vi "Window1.vi"() -> ()   [LabVIEW 8.6]
uses:
  user32.dll
  EventHandlerEnum.ctl
  Engines/SettingsEngine/SettingsEngineEnum.ctl
  <vilib>/Instr/_visa.llb/VISA Set IO Buffer Mask.ctl
  <vilib>/Instr/_visa.llb/VISA Configure Serial Port (Instr).vi
panel:
  in  "Tab Control":enum32{"Main", "Setup", "Debug Data"}(tab)
  in  "FPV View":bool
  out "Climb Rate":sgl(knob) scale=-5.0..5.0 scale format="%#.2g"
  out "Course/Bearing":cluster{i16, i16}(knob) scale=0.0..360.0 scale format="%.0f°"
  out "Altitude":cluster{i32, i32}(knob) scale=0.0..200.0
  out "Air Speed":cluster{i16, i16}(knob)={0, 31} scale=0.0..40.0
  out "UAV Longitude 2":dbl format="%.6g°"
  out "Est Time Left":i32
  out "Current WP":i32
  out "Amps":i32
  out "Watts":i32
  out "Throttle":dbl(slide) scale=0.0..100.0
  out "Battery":dbl(slide) scale=0.0..10.0
  out "Pitch":i32
  out "Roll":i32
  out "Nav Display":picture
  out "Distance to WP":i32 format="%.0f m"
  out "Ground Speed":i32 format="%.0f m/s"
  out "Air Speed":i32 format="%.0f m/s"
  out "UAV Longitude":dbl format="%.6g°"
  out "UAV Latitude":dbl format="%.6g°"
  in  "Stop":bool
  in  "WebBrowser":refnum<k7>(container)
  out "StreamingProgressPercentage":i32(slide) scale=0.0..100.0
  out "Baud Rate":string(combo)="9600"
  out "COM Port":refnum<visa-resource-name>
  out "Camera Position 2":T1
  out "Version":string
  out "VersionAppType":i32(ring) items=["EnterpriseClientGE", "ProGE", "PlusGE", "FreeGE", "UnknownGE"]
  out "ElevationExaggeration":dbl
  in  "Set":bool
  in  "AutoPilotSpeed":dbl=0.5
  in  "Camera Position":T2={"Azimuth"=0.0, "FocusPointAltitude"=0.0, "altMode"=1, "FocusPointLatitude"=0.0, "FocusPointLongitude"=0.0, "Range"=0.0, "Tilt"=0.0} {"altMode" items=["RelativeToGroundAltitudeGE", "AbsoluteAltitudeGE"]}
  out "Debug Output":string
  in  "error in":errorcluster
  in  "EARTHLib.IApplicationGE 2":refnum<k7>
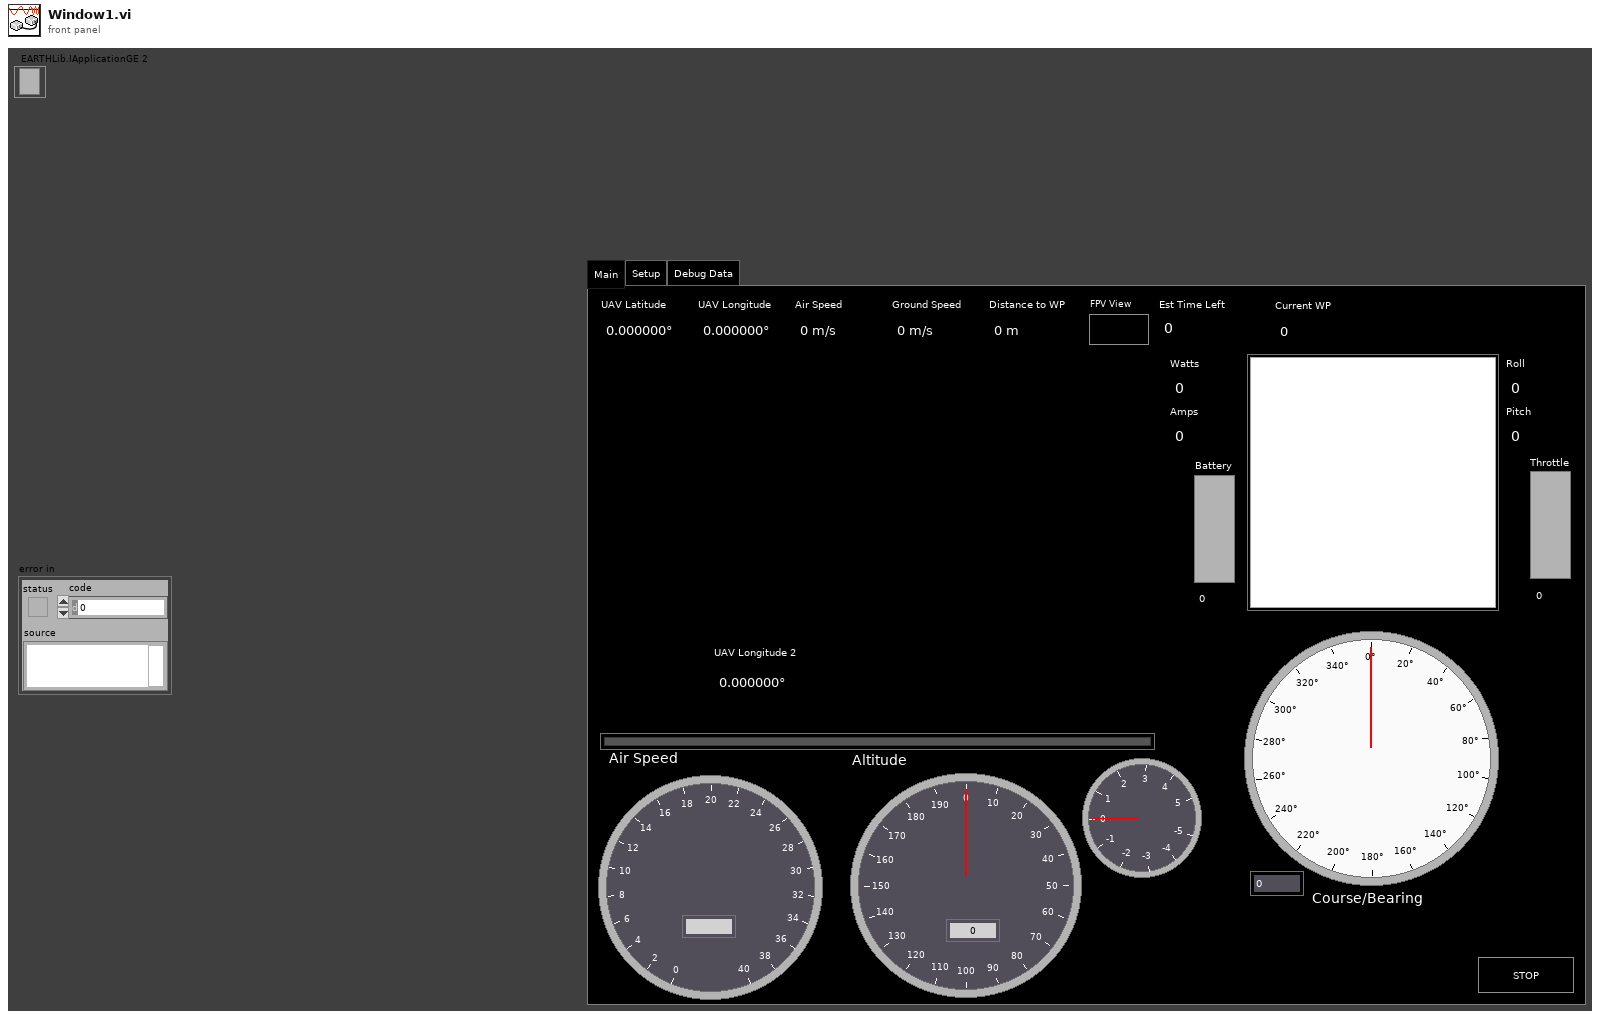
[diagram p1: front panel]
types:
  T1 = cluster{"Azimuth":dbl, "FocusPointAltitude":dbl, "FocusPointAltitudeMode":i32, "FocusPointLatitude":dbl, "FocusPointLongitude":dbl, "Range":dbl, "Tilt":dbl}
  T2 = cluster{"Azimuth":dbl, "FocusPointAltitude":dbl, "altMode":i32, "FocusPointLatitude":dbl, "FocusPointLongitude":dbl, "Range":dbl, "Tilt":dbl}
  T3 = typedef "SettingsEngineEnum.ctl" = enum16{"Init", "Load Settings from File", "Get Setting", "Set/Create Setting", "Save Settings to File"}
  T4 = typedef "VISA Set IO Buffer Mask.ctl" = u16
  T5 = typedef "EventHandlerEnum.ctl" = enum16{"Timeout", "Stop", "UpdateGEView", "UpdateCamData", "FPV_View_On", "UpdateIndicators"}
  T6 = typedef "imagedata.ctl" = cluster{"image type":i32, "image depth":i32, "image":u8[], "mask":u8[], "colors":u32[], "Rectangle":cluster{"left":i16, "top":i16, "right":i16, "bottom":i16}}
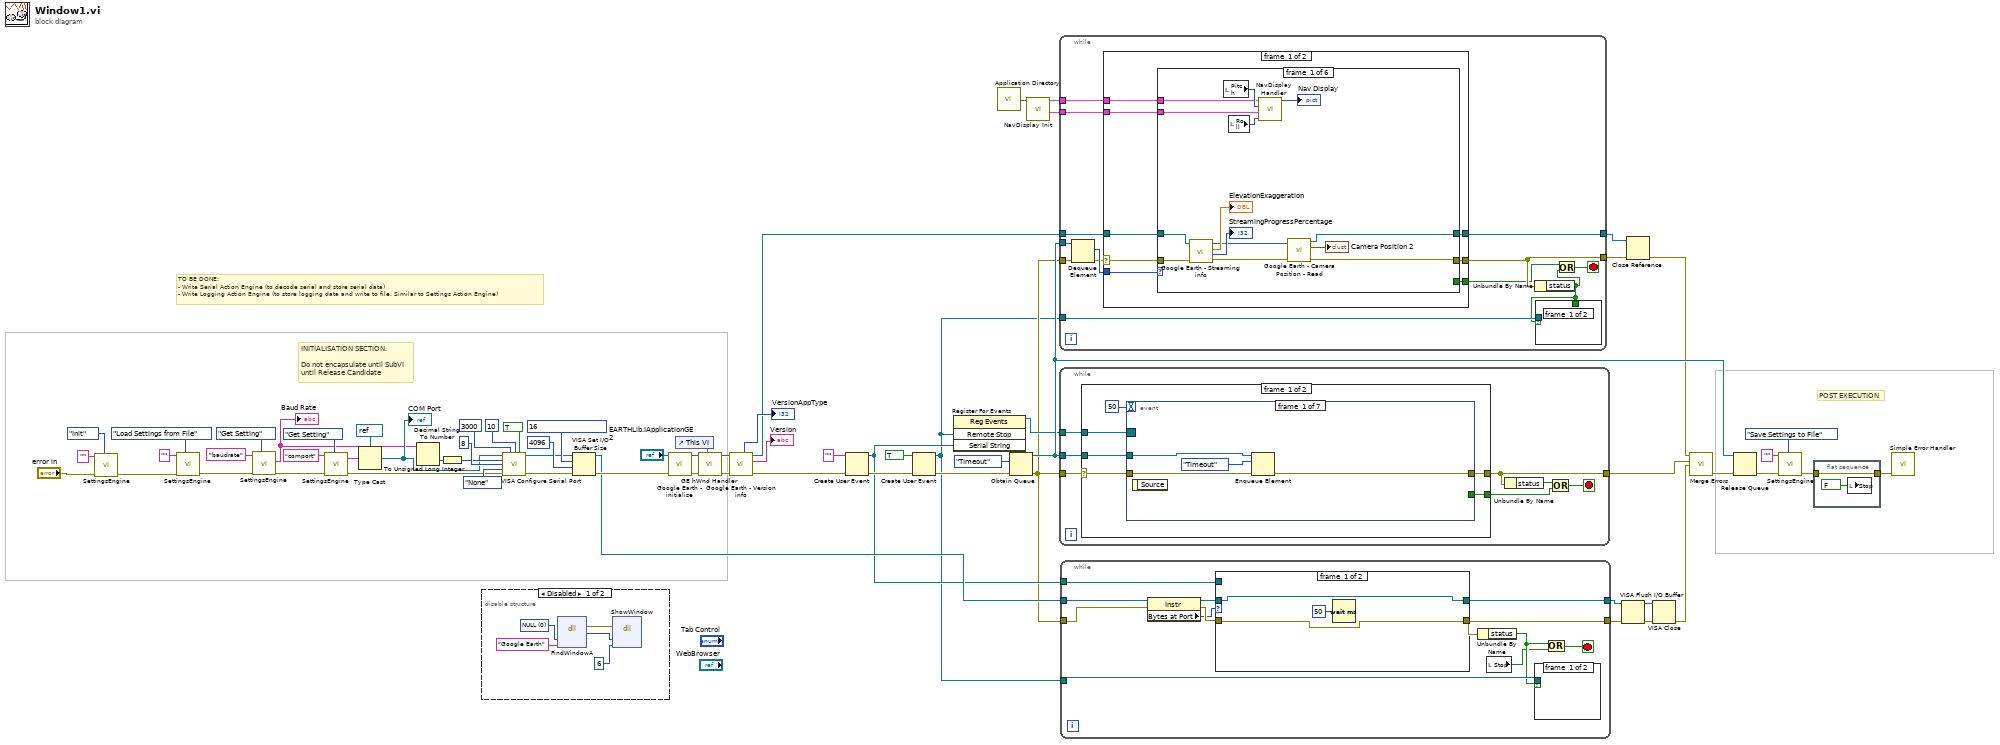
[diagram p0: block diagram]
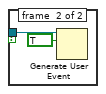
[diagram p2: hidden frame]
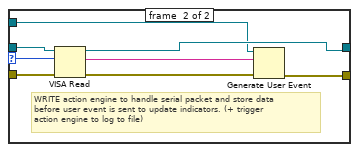
[diagram p3: hidden frame]
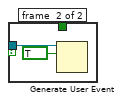
[diagram p4: hidden frame]
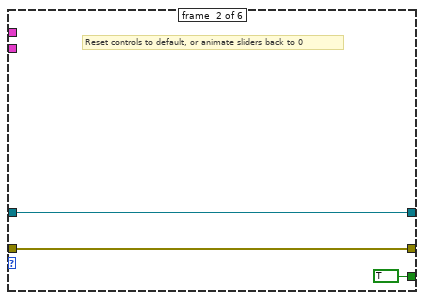
[diagram p5: hidden frame]
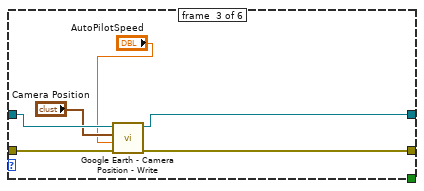
[diagram p6: hidden frame]
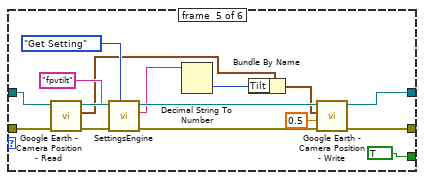
[diagram p8: hidden frame]
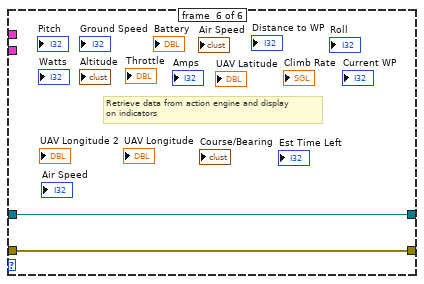
[diagram p9: hidden frame]
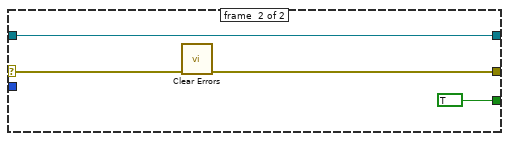
[diagram p10: hidden frame]
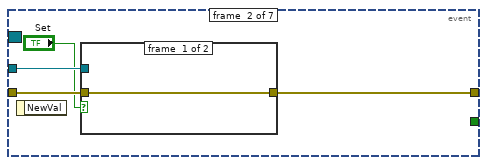
[diagram p11: hidden frame]
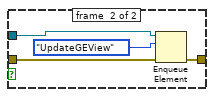
[diagram p12: hidden frame]
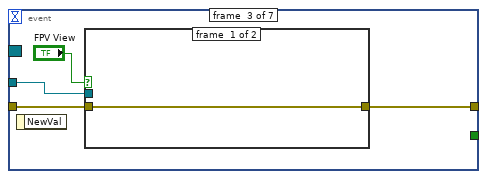
[diagram p13: hidden frame]
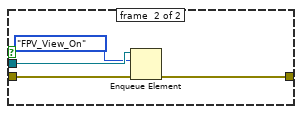
[diagram p14: hidden frame]
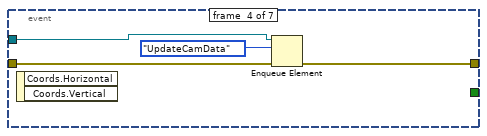
[diagram p15: hidden frame]
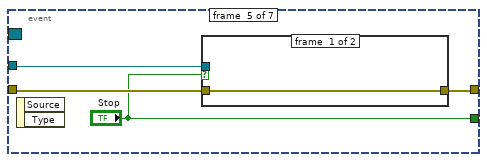
[diagram p16: hidden frame]
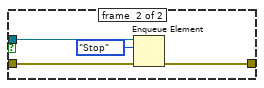
[diagram p17: hidden frame]
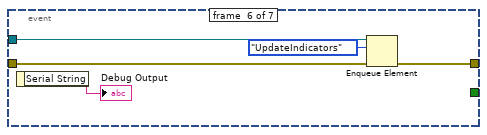
[diagram p18: hidden frame]
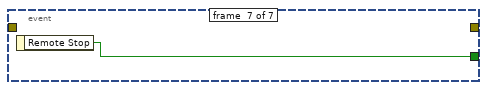
[diagram p19: hidden frame]
diagram:
  w50 = T4 16 items=["I/O Receive Buffer", "I/O Transmit Buffer", "I/O Receive and Transmit Buffer"] ("Mask")
  # "POST EXECUTION"
  # "INITIALISATION SECTION.\n\nDo not encapsulate until SubVI \nuntil Release Candidate"
  # "TO BE DONE:\n- Write Serial Action Engine (to decode serial and store serial data)\n- Write Logging Action Engine (to store logging data and write to file. Similar to Settings Action Engine)"
  n1 = call "SettingsEngine.vi"("Enum"=SettingsEngineEnum."Init", "error in"="error in", "Setting Name"="") -> ("error out"=w3:errorcluster)  [unwired: 7 in, 1 out]
  n2 = call "SettingsEngine.vi"("Enum"=SettingsEngineEnum."Load Settings from File", "error in"=w3, "Setting Name"="") -> ("error out"=w29:errorcluster)  [unwired: 7 in, 1 out]
  n3 = call "SettingsEngine.vi"("Enum"=SettingsEngineEnum."Get Setting", "error in"=w29, "Setting Name"="baudrate") -> ("error out"=w30:errorcluster, "Setting Value"=w5:string)  [unwired: 7 in]
  "Baud Rate" <- w5
  n4 = call "SettingsEngine.vi"("Enum"=SettingsEngineEnum."Get Setting", "error in"=w30, "Setting Name"="comport") -> ("error out"=w38:errorcluster, "Setting Value"=w35:string)  [unwired: 7 in]
  n5 = Type Cast(type=refnum<visa-resource-name> refnum ("VISA resource name"), x=w35) -> (*(type *) &x=w33:refnum<visa-resource-name>)
  "COM Port" <- w33
  n6 = Decimal String To Number(string=w5) -> (number=w42:i32)  [unwired: 3 out]
  n7 = To Unsigned Long Integer(number=w42) -> (unsigned 32bit integer=w41:u32)
  n8 = disable-structure shown="Disabled" {
    frame #0 {
      w73 = 0 items=["NULL"]
      n9 = dll-call lib="user32.dll" fn="FindWindowA" label="FindWindow"("lpszClassName"=w73, "lpszWindowName"="Google Earth") -> (error out=w72:errorcluster, "hWnd"=w70:u32)  [unwired: 4 in, 2 out]
      n10 = dll-call lib="user32.dll" fn="ShowWindow"(error in=w72, "hWnd"=w70, "nCmdShow"=u32 6) -> ()  [unwired: 3 in, 4 out]
    }
    frame #1 {
    }
  }
  n11 = call-poly "VISA Configure Serial Port"("VISA resource name"=w33, "timeout (10sec)"=u32 3000, "termination char\n(0xA = '\\n' = LF)"=u8 10 ("termination char\n(0xA = '\\n' = LF)"), "Enable Termination\nChar (T)"=TRUE ("Enable Termination\nChar (T)"), "baud rate (9600)"=w41, "data bits (8)"=u16 8, "parity (0:none)"=enum16{"None", "Odd", "Even", "Mark", "Space"}."None", "error in (no error)"=w38) -> ("VISA resource name out"=w43:refnum<visa-resource-name>, "error out"=w40:errorcluster)  [unwired: 1 in, 5 out]
  n12 = VISA Set I/O Buffer Size(VISA resource name=w43, mask (16)=w50, size (4096)=u32 4096, error in (no error)=w40) -> (VISA resource name out=w22:refnum<visa-resource-name>, error out=w39:errorcluster)
  n13 = call "Google Earth - initialise.vi"("error in (no error)"=w39, "EARTHLib.IApplicationGE"="EARTHLib.IApplicationGE 2") -> ("error out"=w58:errorcluster, "Refnum Out"=w57:refnum<k7>)  [unwired: 7 in, 1 out]
  n14 = control-ref of="This VI"() -> (w65:refnum<vi>)
  n15 = call "GE hWnd Handler.vi"("This VI"=w65, "error in"=w58, "Refnum In"=w57) -> ("error out"=w66:errorcluster, "Refnum Out"=w59:refnum<k7>)  [unwired: 7 in]
  n16 = call "Google Earth - Version info.vi"("error in"=w66, "Refnum In"=w59) -> ("error out"=w20:errorcluster, "Version"=→"Version":string, "Refnum Out"=w63:refnum<k7>, "VersionAppType"=→"VersionAppType":i32)  [unwired: 6 in]
  n17 = Create User Event(user event datatype="" ("Serial String"), error in=w20) -> (user event=w17:refnum<user-event>, error out=w19:errorcluster)
  n18 = Create User Event(user event datatype=TRUE ("Remote Stop"), error in=w19) -> (user event=w15:refnum<user-event>, error out=w26:errorcluster)
  n19 = register-events(w15, w17) -> (reference out=w25:refnum<event-registration>)  [unwired: 2 in, 1 out]
  n20 = call <vilib>:"Application Directory.vi"() -> ("Application Directory"=w56:path)
  n21 = Obtain Queue(element data type=EventHandlerEnum."Timeout" ("Enum"), error in (no error)=w26) -> (queue out=w67:refnum<queue>, error out=w16:errorcluster)  [unwired: 3 in, 1 out]
  n22 = call "NavDisplay Init.vi"("Application Directory"=w56) -> ("roll image"=w23:T6, "pitch image"=w55:T6)  [unwired: 8 in]
  n23 = while {
    tunnel: w67 -> [w86]
    tunnel: [w79] -> w10
    tunnel: w63 -> [w84]
    tunnel: [w83] -> w60
    tunnel: w23 -> [w81]
    tunnel: w55 -> [w80]
    tunnel: w15 -> [w77]
    tunnel: w16 -> [w75]
    stop <- w76 stop-if-true
    n24 = Dequeue Element(queue=w86, error in (no error)=w75) -> (element=w85:T5, error out=w82:errorcluster)  [unwired: 1 in, 2 out]
    n25 = case shown="No Error" w82 {
      selector: w82 -> [w94 w142]
      tunnel: w85 -> [w96 _]
      tunnel: w84 -> [w95 w141]
      tunnel: [w93 w140] -> w79
      tunnel: [w92 w141] -> w83
      tunnel: w80 -> [w91 _]
      tunnel: w81 -> [w90 _]
      tunnel: [w89 TRUE ("x")] -> w78
      frame #0 {
        n26 = case shown="\"UpdateIndicators\"" w96 {
          tunnel: w95 -> [w108 w113 w119 w121 w134 w137]
          tunnel: w94 -> [w97 w112 w118 w120 w136 w138]
          tunnel: [w98 w112 w116 w120 w135 w138] -> w93
          tunnel: [w100 w113 w115 w121 w132 w137] -> w92
          tunnel: w91 -> [w104 _ _ _ _ _]
          tunnel: w90 -> [w103 _ _ _ _ _]
          tunnel: [_ TRUE ("x") _ _ TRUE ("x") _] -> w89
          frame #0 {
            n27 = call "Google Earth - Streaming info.vi"("error in"=w97, "Refnum in"=w108) -> ("error out"=w99:errorcluster, "StreamingProgressPercentage"=→"StreamingProgressPercentage":i32, "ElevationExaggeration"=→"ElevationExaggeration":dbl, "Refnum Out"=w101:refnum<k7>)  [unwired: 5 in, 1 out]
            n28 = local read "Pitch"() -> (w106:i32)
            n29 = local read "Roll"() -> (w107:i32)
            n30 = call "NavDisplay Handler.vi"("Roll"=w107, "roll image"=w103, "Pitch"=w106, "pitch image"=w104) -> ("new picture"=→"Nav Display":picture)  [unwired: 6 in]
            n31 = call "Google Earth - Camera Position - Read.vi"("error in"=w99, "Refnum in"=w101) -> ("error out"=w98:errorcluster, "Camera Position"=→"Camera Position 2":T1, "Refnum Out"=w100:refnum<k7>)  [unwired: 7 in]
          }
          frame #1 {
            # "Reset controls to default, or animate sliders back to 0"
          }
          frame #2 {
            n32 = call "Google Earth - Camera Position - Write.vi"("error in"=w118, "speed"="AutoPilotSpeed", "Camera Position"="Camera Position", "Refnum in"=w119) -> ("error out"=w116:errorcluster, "Refnum Out"=w115:refnum<k7>)  [unwired: 6 in]
          }
          frame #3 {
          }
          frame #4 {
            n33 = call "Google Earth - Camera Position - Read.vi"("error in"=w136, "Refnum in"=w134) -> ("error out"=w131:errorcluster, "Camera Position"=w123:T1, "Refnum Out"=w133:refnum<k7>)  [unwired: 7 in]
            n34 = call "SettingsEngine.vi"("Enum"=SettingsEngineEnum."Get Setting", "error in"=w131, "Setting Name"="fpvtilt") -> ("error out"=w130:errorcluster, "Setting Value"=w127:string)  [unwired: 7 in]
            n35 = Decimal String To Number(string=w127) -> (number=w126:i32)  [unwired: 2 in, 1 out]
            n36 = Bundle By Name(cluster=w123, "Tilt"=w126) -> (w124:T1)
            n37 = call "Google Earth - Camera Position - Write.vi"("error in"=w130, "speed"=0.5, "Camera Position"=w124, "Refnum in"=w133) -> ("error out"=w135:errorcluster, "Refnum Out"=w132:refnum<k7>)  [unwired: 6 in]
          }
          frame #5 {
            # "Retrieve data from action engine and display\non indicators"
          }
        }
      }
      frame #1 {
        n38 = call <vilib>:"Clear Errors.vi"("error in (no error)"=w142) -> ("error out"=w140:errorcluster)  [unwired: 6 in]
      }
    }
    n39 = Unbundle By Name(w79) -> ("status"=w74:bool)
    n40 = case shown="True" w74 {
      tunnel: w77 -> [_ w88]
      tunnel: w74 -> [_ _]
      frame #0 {
      }
      frame #1 {
        n41 = Generate User Event(user event=w88, event data cluster=TRUE ("event data")) -> ()  [unwired: 1 in, 2 out]
      }
    }
    n42 = Or(x=w78, y=w74) -> (x .or. y?=w76:bool)
  }
  n43 = while {
    tunnel: w67 -> [w149]
    tunnel: w16 -> [w144]
    tunnel: [w147] -> w14
    tunnel: w25 -> [w143]
    stop <- w145 stop-if-true
    n44 = case shown="No Error" w144 {
      selector: w144 -> [w151 w197]
      tunnel: w149 -> [w155 _]
      tunnel: [w153 w197] -> w147
      tunnel: [w152 _] -> w146
      tunnel: w143 -> [w150 _]
      frame #0 {
        n45 = event shown="[5] <Serial String>: User Event" {
          selector: w150 -> [_ _ _ _ _ _ _]
          dyn-events: _ -> [_ _ _ _ _ _ _]
          timeout: 50 -> [_ _ _ _ _ _ _]
          tunnel: w155 -> [w159 w162 w169 w180 w183 w194 _]
          tunnel: w151 -> [w158 w163 w171 w179 w185 w195 _]
          tunnel: [w157 w161 w170 w178 w184 w192 _] -> w153
          tunnel: [_ _ _ _ "Stop" _ w196] -> w152
          event #0 {
            n46 = event-data() -> ()  [unwired: 1 in, 1 out]
            n47 = Enqueue Element(queue=w159, element=EventHandlerEnum."Timeout", error in (no error)=w158) -> (error out=w157:errorcluster)  [unwired: 1 in, 2 out]
          }
          event #1 {
            n48 = event-data() -> ()  [unwired: 1 in, 1 out]
            n49 = case shown="True" "Set" {
              tunnel: w163 -> [w164 w167]
              tunnel: w162 -> [_ w165]
              tunnel: [w164 w166] -> w161
              frame #0 {
              }
              frame #1 {
                n50 = Enqueue Element(queue=w165, element=EventHandlerEnum."UpdateGEView", error in (no error)=w167) -> (error out=w166:errorcluster)  [unwired: 1 in, 2 out]
              }
            }
          }
          event #2 {
            n51 = event-data() -> ()  [unwired: 1 in, 1 out]
            n52 = case shown="True" "FPV View" {
              tunnel: w171 -> [w173 w177]
              tunnel: [w173 w176] -> w170
              tunnel: w169 -> [_ w175]
              frame #0 {
              }
              frame #1 {
                n53 = Enqueue Element(queue=w175, element=EventHandlerEnum."FPV_View_On", error in (no error)=w177) -> (error out=w176:errorcluster)  [unwired: 1 in, 2 out]
              }
            }
          }
          event #3 {
            n54 = event-data() -> ()  [unwired: 1 in, 2 out]
            n55 = Enqueue Element(queue=w180, element=EventHandlerEnum."UpdateCamData", error in (no error)=w179) -> (error out=w178:errorcluster)  [unwired: 1 in, 2 out]
          }
          event #4 {
            n56 = event-data() -> ()  [unwired: 1 in, 2 out]
            n57 = case shown="True" "Stop" {
              tunnel: w185 -> [w186 w190]
              tunnel: [w186 w189] -> w184
              tunnel: w183 -> [_ w188]
              frame #0 {
              }
              frame #1 {
                n58 = Enqueue Element(queue=w188, element=EventHandlerEnum."Stop", error in (no error)=w190) -> (error out=w189:errorcluster)  [unwired: 1 in, 2 out]
              }
            }
          }
          event #5 {
            n59 = event-data() -> ("Serial String"=→"Debug Output":string)  [unwired: 1 in]
            n60 = Enqueue Element(queue=w194, element=EventHandlerEnum."UpdateIndicators", error in (no error)=w195) -> (error out=w192:errorcluster)  [unwired: 1 in, 2 out]
          }
          event #6 {
            n61 = event-data() -> ("Remote Stop"=w196:bool)  [unwired: 1 in]
          }
        }
      }
      frame #1 {
      }
    }
    n62 = Unbundle By Name(w147) -> ("status"=w148:bool)
    n63 = Or(x=w148, y=w146) -> (x .or. y?=w145:bool)
  }
  n64 = while {
    tunnel: w22 -> [w208]
    tunnel: [w209] -> w21
    tunnel: w17 -> [w204]
    tunnel: w16 -> [w203]
    tunnel: [w201] -> w12
    tunnel: w15 -> [w202]
    stop <- w200 stop-if-true
    n65 = property class="Instr"(reference=w208, error in=w203) -> (reference out=w207:refnum<visa-resource-name>, error out=w206:errorcluster, "Bytes at Port"=w205:u32)
    n66 = case shown="200" w205 {
      selector: w205 -> [_ w219]
      tunnel: [w212 w222] -> w209
      tunnel: w207 -> [w212 w221]
      tunnel: w206 -> [w213 w220]
      tunnel: w204 -> [_ w216]
      tunnel: [w213 w215] -> w201
      frame #0 {
        n67 = Wait (ms)(milliseconds to wait=u32 50) -> ()  [unwired: 1 out]
      }
      frame #1 {
        # "WRITE action engine to handle serial packet and store data\nbefore user event is sent to update indicators. (+ trigger\naction engine to log to file)"
        n68 = VISA Read(VISA resource name=w221, byte count=w219, error in (no error)=w220) -> (VISA resource name out=w222:refnum<visa-resource-name>, read buffer=w217:string, error out=w218:errorcluster)  [unwired: 1 out]
        n69 = Generate User Event(user event=w216, event data cluster=w217, error in=w218) -> (error out=w215:errorcluster)  [unwired: 1 out]
      }
    }
    n70 = Unbundle By Name(w201) -> ("status"=w199:bool)
    n71 = local read "Stop"() -> (w198:bool)
    n72 = case shown="True" w199 {
      tunnel: w202 -> [_ w211]
      frame #0 {
      }
      frame #1 {
        n73 = Generate User Event(user event=w211, event data cluster=TRUE ("event data")) -> ()  [unwired: 1 in, 2 out]
      }
    }
    n74 = Or(x=w199, y=w198) -> (x .or. y?=w200:bool)
  }
  n75 = VISA Flush I/O Buffer(VISA resource name=w21, error in (no error)=w12) -> (VISA resource name out=w28:refnum<visa-resource-name>, error out=w27:errorcluster)  [unwired: 1 out]
  n76 = Close Reference(reference=w60, error in (no error)=w10) -> (error out=w9:errorcluster)
  n77 = VISA Close(VISA resource name=w28, error in (no error)=w27) -> (error out=w11:errorcluster)
  n78 = call <vilib>:"Merge Errors.vi"("error in 3 (no error)"=w11, "error in 2 (no error)"=w14, "error in 1 (no error)"=w9) -> ("error out"=w13:errorcluster)  [unwired: 4 in]
  n79 = Release Queue(queue=w67, error in (no error)=w13) -> (error out=w8:errorcluster)  [unwired: 1 in, 2 out]
  n80 = call "SettingsEngine.vi"("Enum"=SettingsEngineEnum."Save Settings to File", "error in"=w8, "Setting Name"="") -> ("error out"=w6:errorcluster)  [unwired: 7 in, 1 out]
  n81 = flat-sequence {
    tunnel: [w223] -> w7
    tunnel: w6 -> [w223]
    frame #0 {
      n82 = local write "Stop"(FALSE ("Stop")) -> ()
    }
  }
  n83 = call <vilib>:"Simple Error Handler.vi"("error in (no error)"=w7) -> ()  [unwired: 4 in, 5 out]
